vi "Add Item.vi"(8 "error in (no error)":errorcluster caption="错误输入（无错误）", 10 "ItemRef":refnum<k24>, 11 "StatusStripClass 输入":refnum<class "StatusStripClass.lvclass"> caption="DNL_LabVIEW Object in") -> (0 "error out":errorcluster caption="错误输出", 3 "StatusStripClass 输出":refnum<class "StatusStripClass.lvclass"> caption="DNL_LabVIEW Object out")   [LabVIEW 2013, in "StatusStripClass.lvclass"]
uses:
  StatusStripClass.lvclass
  System.Windows.Forms
  StatusStripClass.lvclass/StatusStripClass.ctl
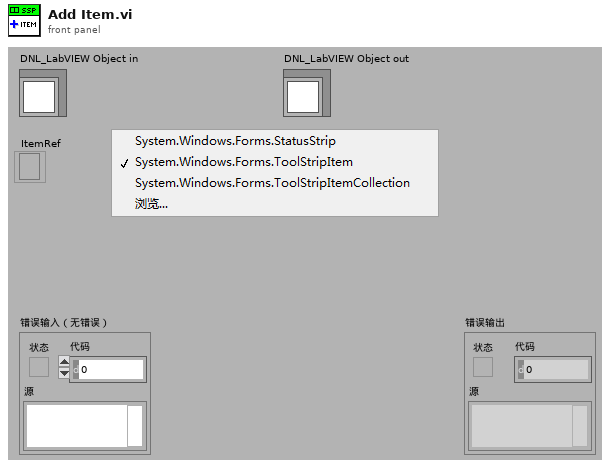
[diagram p1: front panel]
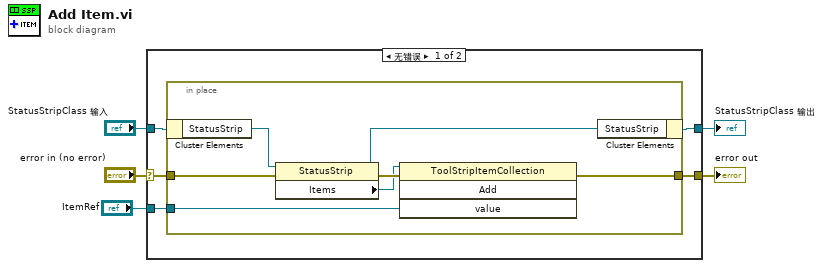
[diagram p0: block diagram]
diagram:
  n1 = case shown="无错误" "error in (no error)" {
    selector: "error in (no error)" -> [w7 w19]
    tunnel: [w10 w19] -> w4
    tunnel: [w8 w18] -> w2
    tunnel: "StatusStripClass 输入" -> [w9 w18]
    tunnel: "ItemRef" -> [w6 _]
    frame No Error {
      n2 = in-place {
        in-place-border: [w15] -> w10
        in-place-border: w6 -> [w12]
        in-place-border: w7 -> [w11]
        n3 = in-place-cluster #1(w9) -> ("StatusStrip"=w14:refnum<k24>)
        n4 = property class="StatusStrip"(reference=w14, error in=w11) -> (reference out=w13:refnum<k24>, error out=w17:errorcluster, "Items"=w16:refnum<k24>)
        n5 = invoke class="ToolStripItemCollection" method="Add"(reference=w16, error in=w17, "value"=w12) -> (error out=w15:errorcluster)  [unwired: 1 in, 3 out]
        n6 = in-place-cluster #1("StatusStrip"=w13) -> (w8:refnum<class "StatusStripClass.lvclass">)
      }
    }
    frame Error {
    }
  }
  "error out" <- w4
  "StatusStripClass 输出" <- w2
